vi "Untitled 2.vi"() -> ()   [LabVIEW 2017]
uses:
  MARLIN.lvclass
panel:
  in  "Numeric":dbl
  out "MARLIN.lvclass 2":refnum<class "MARLIN.lvclass">
  in  "MARLIN.lvclass":refnum<class "MARLIN.lvclass">
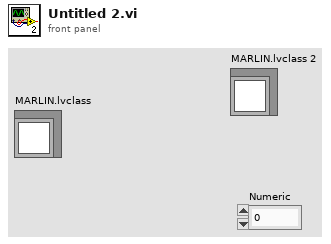
[diagram p1: front panel]
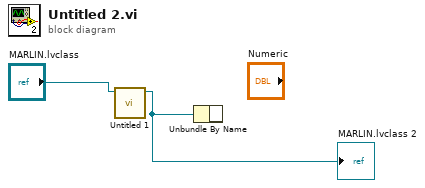
[diagram p0: block diagram]
diagram:
  n1 = call-dynamic "Untitled 1.vi"("MARLIN in"="MARLIN.lvclass") -> ("MARLIN out"=w1:refnum<class "MARLIN.lvclass">)  [unwired: 9 in, 1 out]
  "MARLIN.lvclass 2" <- w1
  n2 = Unbundle By Name(w1) -> ()  [unwired: 1 out]
